vi "GetTextFromStrCtrl.vi"(11 "string ref":refnum<vi>) -> (3 "string out":string)   [LabVIEW 2018, in "Library-Ctrl.lvlib"]
uses:
  Library-Ctrl.lvlib
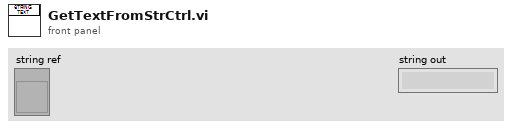
[diagram p1: front panel]
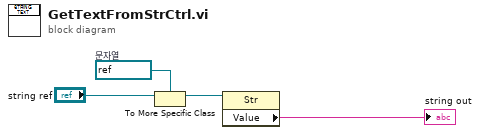
[diagram p0: block diagram]
diagram:
  w3 = refnum<vi> refnum  # 문자열
  n1 = To More Specific Class(target class=w3, reference="string ref") -> (specific class reference=w2:refnum<vi>)  [unwired: 1 in, 1 out]
  n2 = property class="Str"(reference=w2) -> ("Value"=→"string out":string)  [unwired: 1 in, 2 out]
